vi "LinearAndAngularProfileGenerator.vi"(0 "Radius":dbl=200.0, 1 "MaxVelAngular":dbl=100.0, 2 "MaxAccelAngular":dbl=100.0, 5 "Theta":dbl=200.0, 7 "InitialVelocity":dbl, 9 "FinalVelocity":dbl, 11 "dt":u32=20, 12 "MaxVelocity":dbl=100.0, 13 "MaxAccel":dbl=75.0) -> (4 "Linear":cluster{"Pos":dbl[], "Vel":dbl[]}, 6 "Angular":cluster{"Pos":dbl[], "Vel":dbl[]}, 15 "dt":u32=20)   [LabVIEW 2016]
panel:
  out "Angle":dbl[][](graph)
  out "Linear":dbl[][](graph)
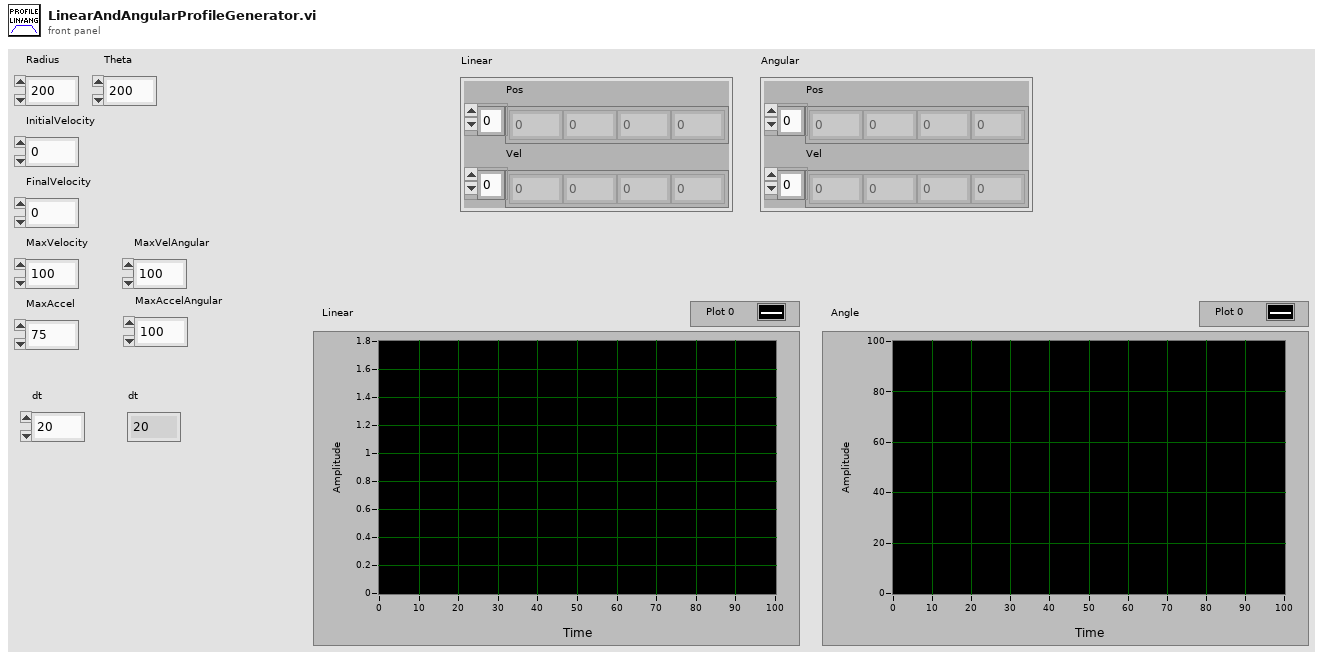
[diagram p1: front panel]
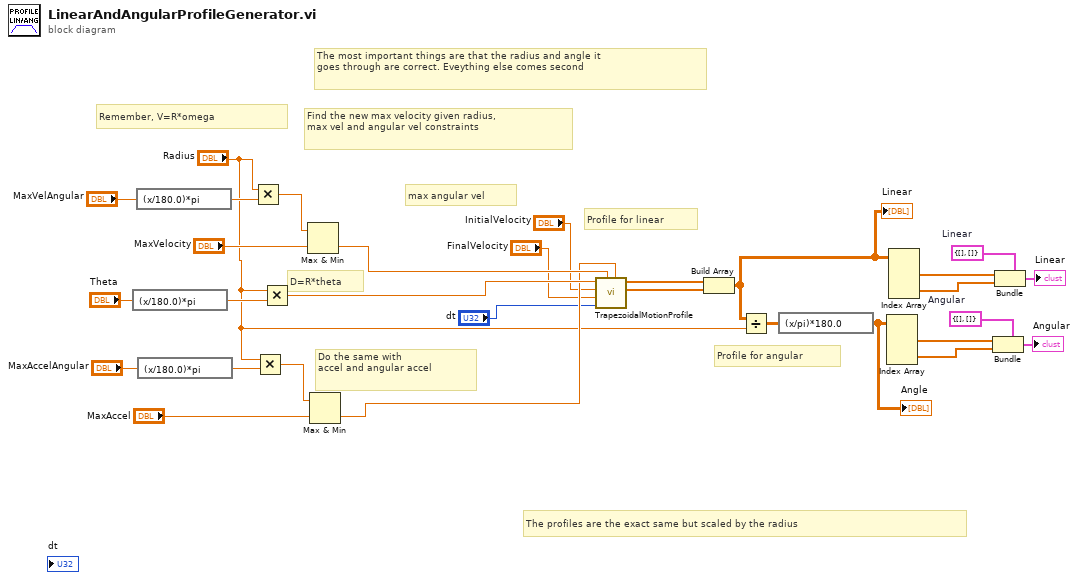
[diagram p0: block diagram]
diagram:
  w5 = cluster{"Pos":dbl[], "Vel":dbl[]} {"Pos"=[], "Vel"=[]}  # Angular
  w8 = cluster{"Pos":dbl[], "Vel":dbl[]} {"Pos"=[], "Vel"=[]}  # Linear
  # "The profiles are the exact same but scaled by the radius"
  # "D=R*theta"
  # "Profile for angular"
  # "Profile for linear"
  # "Do the same with\naccel and angular accel"
  # "max angular vel"
  # "Find the new max velocity given radius, \nmax vel and angular vel constraints"
  # "The most important things are that the radius and angle it \ngoes through are correct. Eveything else comes second"
  # "Remember, V=R*omega"
  n1 = expression code="(x/180.0)*pi" ("degrees to radians")("Theta") -> (w15:dbl)
  n2 = expression code="(x/180.0)*pi" ("degrees to radians")("MaxVelAngular") -> (w18:dbl)
  n3 = expression code="(x/180.0)*pi" ("degrees to radians")("MaxAccelAngular") -> (w19:dbl)
  n4 = Multiply(x="Radius", y=w18) -> (x*y=w30:dbl)
  n5 = Multiply(x="Radius", y=w19) -> (x*y=w28:dbl)
  n6 = Multiply(x="Radius", y=w15) -> (x*y=w26:dbl)
  n7 = Max & Min(x=w30, y="MaxVelocity") -> (min(x,y)=w25:dbl)  [unwired: 1 out]
  n8 = Max & Min(x=w28, y="MaxAccel") -> (min(x,y)=w24:dbl)  [unwired: 1 out]
  n9 = call "TrapezoidalMotionProfile.vi"("MaxAccel"=w24, "MaxVelocity"=w25, "dt"="dt", "FinalVelocity"="FinalVelocity", "InitialVelocity"="InitialVelocity", "Distance"=w26) -> ("Vel"=w21:dbl[], "Pos"=w22:dbl[])  [unwired: 2 in, 2 out]
  n10 = Build Array(w22, w21) -> (w1:dbl[][])
  "Linear" <- w1
  n11 = Divide(x=w1, y="Radius") -> (x/y=w13:dbl[][])
  n12 = expression code="(x/pi)*180.0" ("radians to degrees")(w13) -> (w2:dbl[][])
  "Angle" <- w2
  n13 = Index Array(array=w2) -> (element #1=w3:dbl[], element #2=w4:dbl[])  [unwired: 4 in]
  n14 = Index Array(array=w1) -> (element #1=w10:dbl[], element #2=w9:dbl[])  [unwired: 4 in]
  n15 = Bundle(cluster=w5, "Pos"=w3, "Vel"=w4) -> (→"Angular":cluster{"Pos":dbl[], "Vel":dbl[]})
  n16 = Bundle(cluster=w8, "Pos"=w10, "Vel"=w9) -> (→"Linear":cluster{"Pos":dbl[], "Vel":dbl[]})
